vi "Action Delete Instrument Name.vi"(0 "VISA resource name":refnum<visa-resource-name>, 5 "Logical Instrument Name":string, 11 "error in (no error)":errorcluster) -> (4 "VISA resource name out":refnum<visa-resource-name>, 15 "error out":errorcluster)   [LabVIEW 2012, in "NH Research Regenerative Test Series.lvlib"]
doc: "Disassociates identifier’s from the logical instrument number. After this executes, the default identifier is re-associated with the instrument number.\n\nNOTE: The 4900 only has one logical instrument so the only valid instrument number is 1."
uses:
  <instrlib>/NH Research Regenerative Test Series/NH Research Regenerative Test Series.lvlib
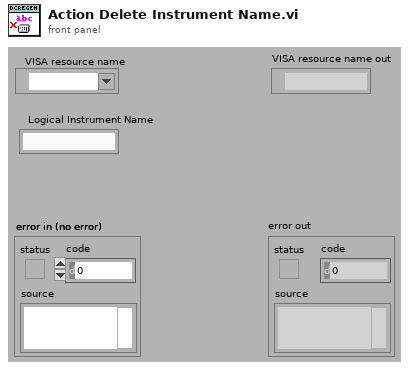
[diagram p1: front panel]
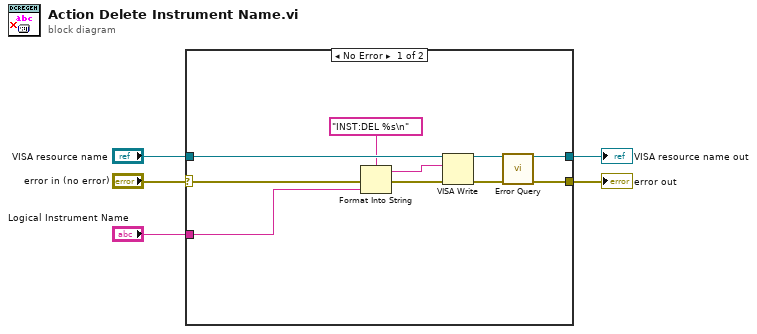
[diagram p0: block diagram]
diagram:
  n1 = case shown="No Error" "error in (no error)" {
    selector: "error in (no error)" -> [w10 w17]
    tunnel: "VISA resource name" -> [w15 w16]
    tunnel: [w12 w16] -> w4
    tunnel: [w11 w17] -> w3
    tunnel: "Logical Instrument Name" -> [w6 _]
    frame No Error {
      n2 = Format Into String(format string="INST:DEL %s\n" ("Command"), error in=w10, w6) -> (resulting string=w13:string, error out=w9:errorcluster)  [unwired: 1 in]
      n3 = VISA Write(VISA resource name=w15, write buffer=w13, error in (no error)=w9) -> (VISA resource name out=w8:refnum<visa-resource-name>, error out=w7:errorcluster)  [unwired: 1 out]
      n4 = call <instrlib>:"Error Query.vi"("VISA resource name"=w8, "error in (no error)"=w7) -> ("VISA resource name out"=w12:refnum<visa-resource-name>, "error out"=w11:errorcluster)  [unwired: 10 in, 2 out]
    }
    frame Error {
    }
  }
  "error out" <- w3
  "VISA resource name out" <- w4
